vi "remove temp folder from config.vi"(11 "Config in":T1) -> (3 "Config out":T1)   [LabVIEW 2023, in "User Interface.lvlib"]
uses:
  User Interface.lvlib
  Controls/configuration cluster.ctl
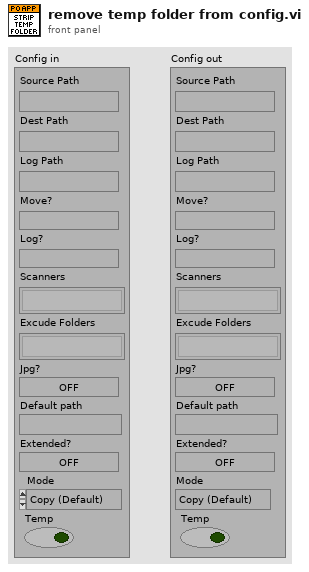
[diagram p1: front panel]
types:
  T1 = typedef "User Interface.lvlib/configuration cluster.ctl" = cluster{"Source Path":path, "Dest Path":path, "Log Path":path, "Move?":bool, "Log?":bool, "Scanners":string[], "Excude Folders":string[], "Jpg?":bool, "Default path":path, "Extended?":bool, "Mode":enum16{"Copy (Default)", "Move", "Rename"}, "Temp":bool}
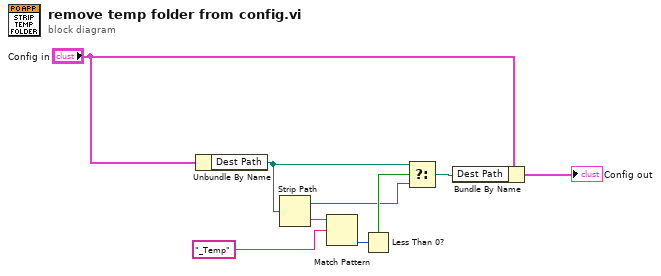
[diagram p0: block diagram]
diagram:
  n1 = Unbundle By Name("Config in") -> ("Dest Path"=w7:path)
  n2 = Strip Path(path=w7) -> (stripped path=w8:path, name=w1:string)
  n3 = Match Pattern(string=w1, regular expression="_Temp") -> (offset past match=w5:i32)  [unwired: 1 in, 3 out]
  n4 = Less Than 0?(x=w5) -> (x < 0?=w9:bool)
  n5 = Select(t=w7, s=w9, f=w8) -> (s? t:f=w6:path)
  n6 = Bundle By Name(cluster="Config in", "Dest Path"=w6) -> (→"Config out":T1)
